vi "G#Debugger_Init.vi"(0 "This VI":refnum<vi>, 5 "error in (no error)":errorcluster) -> (14 "refs":T1, 16 "GUI Event Registration Refnum":refnum<event-registration>, 17 "Application Instance":string, 19 "error out":errorcluster)   [LabVIEW 2017, in "G#Debugger.lvlib"]
uses:
  G#Debugger.lvlib
  G#Debugger_Refs.ctl
  G#Object/utils/G#Object_ClassInfoType.ctl
  G#Object/G#Object.lvclass
  G#Object/utils/G#Object_ObjectInfoType.ctl
  G#Object/utils/G#Object_CreateMethod.ctl
  G#Debugger_SubPanelInfo.ctl
  G#Object/utils/G#Object_ClassHierarchy.ctl
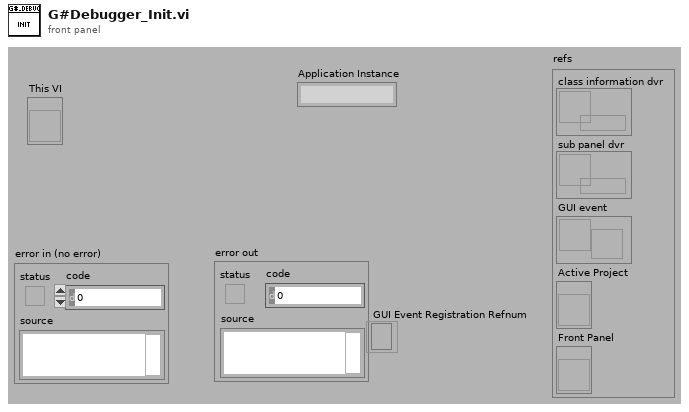
[diagram p1: front panel]
types:
  T1 = typedef "G#Debugger.lvlib/G#Debugger_Refs.ctl" = cluster{"class information dvr":refnum<data-value>, "sub panel dvr":refnum<data-value>, "GUI event":refnum<user-event>, "Active Project":refnum<vi>, "Front Panel":refnum<vi>}
  T2 = typedef "G#Debugger.lvlib/G#Debugger_SubPanelInfo.ctl" = cluster{"Ref":refnum<class "G#Object.lvclass">, "class hierarchy":T3[], "class attributes":path[], "object attributes":path[], "inheritance index":i32, "is class attributes":bool, "vi reference":refnum<vi>}
  T3 = typedef "G#Object.lvclass/G#Object_ClassHierarchy.ctl" = cluster{"ClassName":string, "FullClassName":string, "ClassPath":path, "IsLeaf":bool}
  T4 = typedef "G#Object.lvclass/G#Object_ClassInfoType.ctl" = cluster{"ClassName":string, "ObjectInfo":T5[], "ObjectRefs":refnum<class "G#Object.lvclass">[], "TypeRef":refnum<class "G#Object.lvclass">}
  T5 = typedef "G#Object.lvclass/G#Object_ObjectInfoType.ctl" = cluster{"ObjectName":string, "ObjectID":u32, "Users":i32, "Counter":bool, "AttributeRefs":u32[], "FullClassName":string, "ClassName":string, "CreateMethod":T6, "GenericDestructorExists":bool, "Owner":string}
  T6 = typedef "G#Object.lvclass/G#Object_CreateMethod.ctl" = enum16{"Create", "Create or look up existing", "Look up existing"}
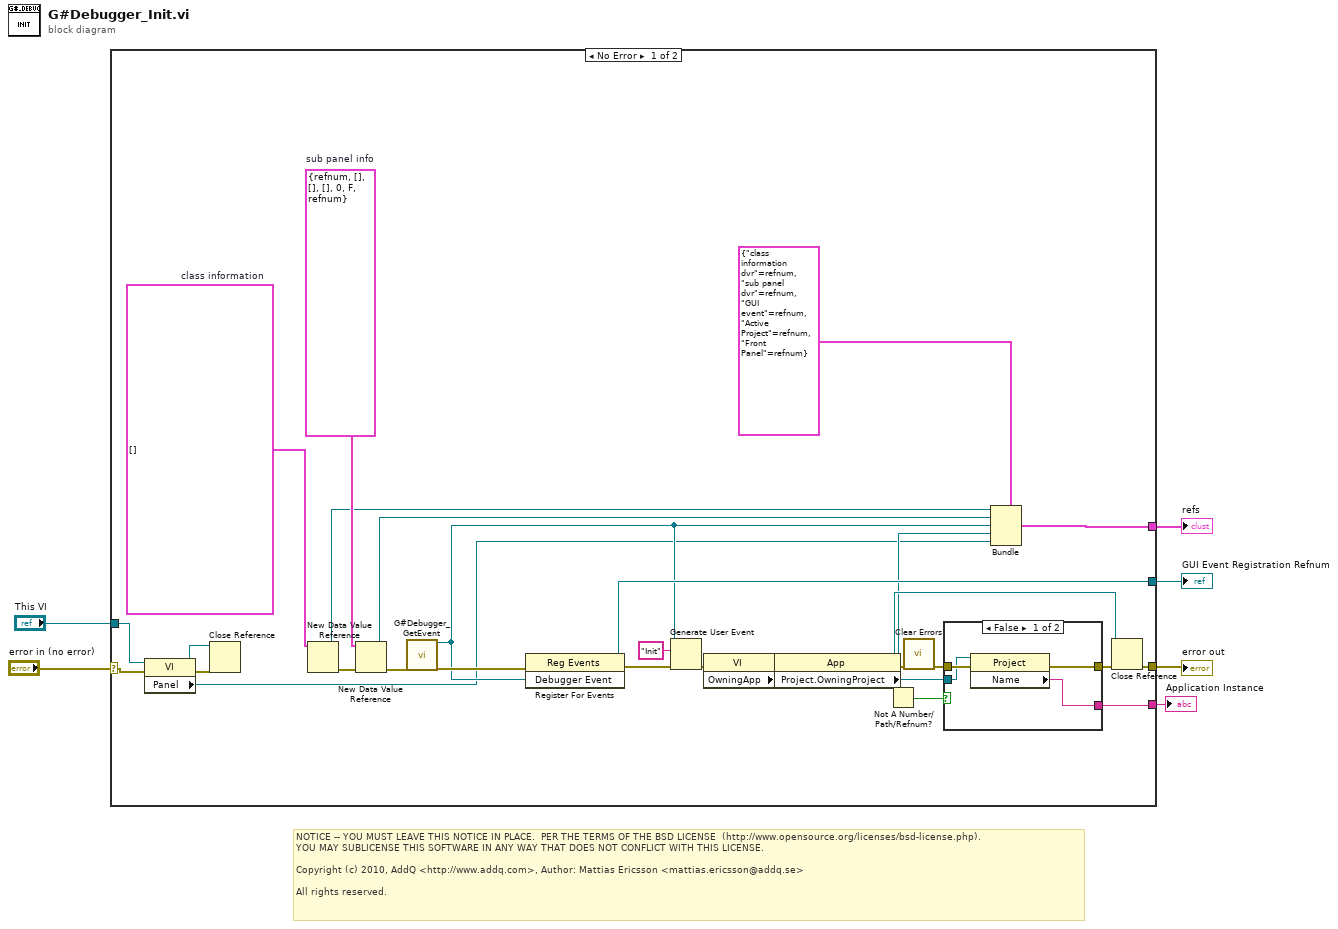
[diagram p0: block diagram]
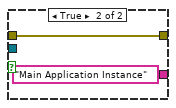
[diagram p2: hidden frame]
diagram:
  # "NOTICE -- YOU MUST LEAVE THIS NOTICE IN PLACE.  PER THE TERMS OF THE BSD LICENSE  (http://www.opensource.org/licenses/bsd-license.php).\nYOU MAY SUBLICENSE THIS SOFTWARE IN ANY WAY THAT DOES NOT CONFLICT WITH THIS LICENSE.\n\nCopyright (c) 2010, AddQ <http://www.addq.com>, Author: Mattias Ericsson <mattias.ericsson@addq.se>\n\nAll rights reserved."
  n1 = case shown="No Error" "error in (no error)" {
    selector: "error in (no error)" -> [w11 w42]
    tunnel: [w19 w42] -> w5
    tunnel: [w29 _] -> w4
    tunnel: [w26 _] -> w3
    tunnel: [w21 _] -> w2
    tunnel: "This VI" -> [w10 _]
    frame No Error {
      w32 = T2 {"Ref"=refnum, "class hierarchy"=[], "class attributes"=[], "object attributes"=[], "inheritance index"=0, "is class attributes"=FALSE, "vi reference"=refnum}  # sub panel info
      w34 = T4[] []  # class information
      n2 = property class="VI"(reference=w10, error in=w11) -> (reference out=w8:refnum<vi>, error out=w9:errorcluster, "Panel"=w7:refnum<vi>)
      n3 = Close Reference(reference=w8, error in (no error)=w9) -> ()  [unwired: 1 out]
      n4 = New Data Value Reference(data value=w34) -> (data value reference=w31:refnum<data-value>, error out=w33:errorcluster)  [unwired: 1 in]
      n5 = New Data Value Reference(data value=w32, error in=w33) -> (data value reference=w30:refnum<data-value>, error out=w16:errorcluster)
      n6 = call "G#Debugger_GetEvent.vi"("error in (no error)"=w16) -> ("Debugger Event"=w14:refnum<user-event>, "error out"=w15:errorcluster)  [unwired: 17 in]
      n7 = register-events(error in=w15, w14) -> (reference out=w26:refnum<event-registration>, error out=w27:errorcluster)  [unwired: 1 in]
      n8 = Generate User Event(user event=w14, event data cluster="Init" ("event data"), error in=w27) -> (error out=w24:errorcluster)  [unwired: 1 in, 1 out]
      n9 = property class="VI"(error in=w24) -> (error out=w23:errorcluster, "OwningApp"=w25:refnum<vi>)  [unwired: 1 in, 1 out]
      n10 = property class="App"(reference=w25, error in=w23) -> (reference out=w18:refnum<vi>, error out=w13:errorcluster, "Project.OwningProject"=w17:refnum<vi>)
      n11 = Not A Number/Path/Refnum?(number/path/refnum=w17) -> (NaN/Path/Refnum?=w22:bool)
      n12 = call <vilib>:"Clear Errors.vi"("error in (no error)"=w13) -> ("error out"=w12:errorcluster)  [unwired: 5 in, 1 out]
      n13 = case shown="False" w22 {
        tunnel: w12 -> [w39 w41]
        tunnel: w17 -> [w38 _]
        tunnel: [w36 w41] -> w20
        tunnel: [w37 "Main Application Instance" ("Name")] -> w21
        frame False {
          n14 = property class="Project"(reference=w38, error in=w39) -> (error out=w36:errorcluster, "Name"=w37:string)  [unwired: 1 out]
        }
        frame True {
        }
      }
      n15 = Bundle(cluster=T1 {"class information dvr"=refnum, "sub panel dvr"=refnum, "GUI event"=refnum, "Active Project"=refnum, "Front Panel"=refnum} ("refs"), "class information dvr"=w31, "sub panel dvr"=w30, "GUI event"=w14, "Active Project"=w17, "Front Panel"=w7) -> (w29:T1)
      n16 = Close Reference(reference=w18, error in (no error)=w20) -> (error out=w19:errorcluster)
    }
    frame Error {
    }
  }
  "error out" <- w5
  "refs" <- w4
  "GUI Event Registration Refnum" <- w3
  "Application Instance" <- w2
